vi "POP send LIST.vi"(3 "error in":errorcluster, 4 "MSG number":i32=-1, 5 "connection ID in":refnum<k5>) -> (0 "error out":errorcluster, 1 "LIST response":string="\r\n", 2 "connection ID out":refnum<k5>)   [LabVIEW 2012]
doc: "This low-level POP VI sends the \"LIST\" command to a mail server, instructing it either to list all messages currently held for the user on the server (an argument less than 0), or to display information about a specific message (an argument from 1 to N, assuming there are N messages stored on the server)."
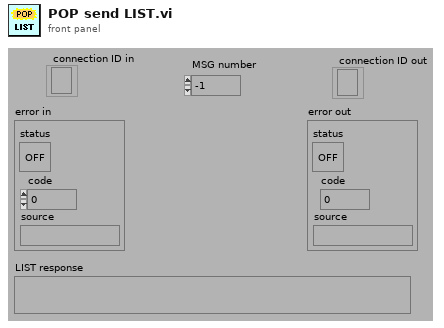
[diagram p1: front panel]
types:
  T1 = enum16{"Standard", "Buffered", "CRLF", "Immediate"}
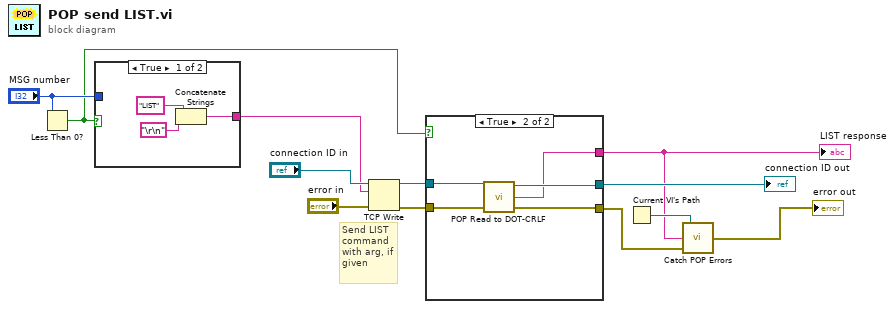
[diagram p0: block diagram]
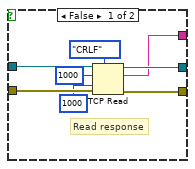
[diagram p2: hidden frame]
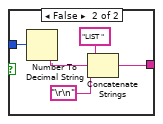
[diagram p3: hidden frame]
diagram:
  # "Send LIST\ncommand\nwith arg, if\ngiven"
  n1 = Less Than 0?(x="MSG number") -> (x < 0?=w5:bool)
  n2 = case shown="True" w5 {
    tunnel: "MSG number" -> [_ w18]
    tunnel: [w13 w16] -> w6
    frame True {
      n3 = Concatenate Strings("LIST", "\r\n") -> (w13:string)
    }
    frame False {
      n4 = Number To Decimal String(number=w18) -> (decimal integer string=w17:string)  [unwired: 1 in]
      n5 = Concatenate Strings("LIST ", w17, "\r\n") -> (w16:string)
    }
  }
  n6 = TCP Write(connection ID="connection ID in", data in=w6, error in (no error)="error in") -> (connection ID out=w12:refnum<k5>, error out=w11:errorcluster)  [unwired: 1 in, 1 out]
  n7 = case shown="True" w5 {
    tunnel: w12 -> [w27 w33]
    tunnel: w11 -> [w26 w32]
    tunnel: [w23 w31] -> w8
    tunnel: [w22 w29] -> w3
    tunnel: [w21 w30] -> w2
    frame False {
      # "Read response"
      n8 = TCP Read(connection ID=w27, bytes to read=1000, error in (no error)=w26, 7:T1."CRLF" ("mode (standard)"), 9:1000 ("timeout ms (25000)")) -> (connection ID out=w23:refnum<k5>, data out=w21:string, error out=w22:errorcluster)
    }
    frame True {
      n9 = call "POP Read to DOT-CRLF.vi"("error in"=w32, "connection ID in"=w33) -> ("error out"=w29:errorcluster, "LIST response"=w30:string, "connection ID out"=w31:refnum<k5>)  [unwired: 1 in]
    }
  }
  "LIST response" <- w2
  "connection ID out" <- w8
  n10 = Current VI's Path() -> (path=w4:path)
  n11 = call "Catch POP Errors.vi"("error in"=w3, "POP server response"=w2, "Caller Path"=w4) -> ("error out"=→"error out":errorcluster)
